vi "RELATORIO2LABVIEW.vi"() -> ()   [LabVIEW 2019]
uses:
  <vilib>/Instr/_visa.llb/VISA Configure Serial Port (Instr).vi
  <vilib>/express/express analysis/Spectral/Block/exnSpectralBlock spectral measurements RMS poly.vi
  <vilib>/express/express analysis/Spectral/Block/exnSpectralBlock spectral measurements RMS WFM.vi
  <vilib>/express/express analysis/Spectral/XNode/ExpressSpectralMeasurementsBlockNode.xnode
panel:
  out "Si":bool
  out "Lá":bool
  out "Sol":bool
  out "Fá":bool
  out "Mi":bool
  out "Ré":bool
  out "Dó":bool
  out "Análise espectral da onda - FFT (RMS)":cluster{"f0":dbl, "df":dbl, "magnitude":dbl[]}(graph)
  out "Amplitude do sinal (v) x tempo (s):":waveform(dbl)(graph)
  in  "Parar":bool
  out "Número de \nAmostras":u32 caption="Número de Amostras"
  in  "Número de Blocos de Dados":u32=100 min=1 max=50000 step=1
  in  "Frequencia de Amostragem":dbl=75000.0
  in  "VCC":dbl=5.0
  in  "Resolução":i16=8
  in  "COM Port":refnum<visa-resource-name>
  in  "Baudrate":u32=2000000
  # "PSI3214 - Turma 6\nAntonio Oliveira Pedroso da Cruz — 11798787\nDaniel Martins Cabanas — 12486742\nJoão Pedro Lima A. de Carvalho — 11260846"
  # "Notas musicais"
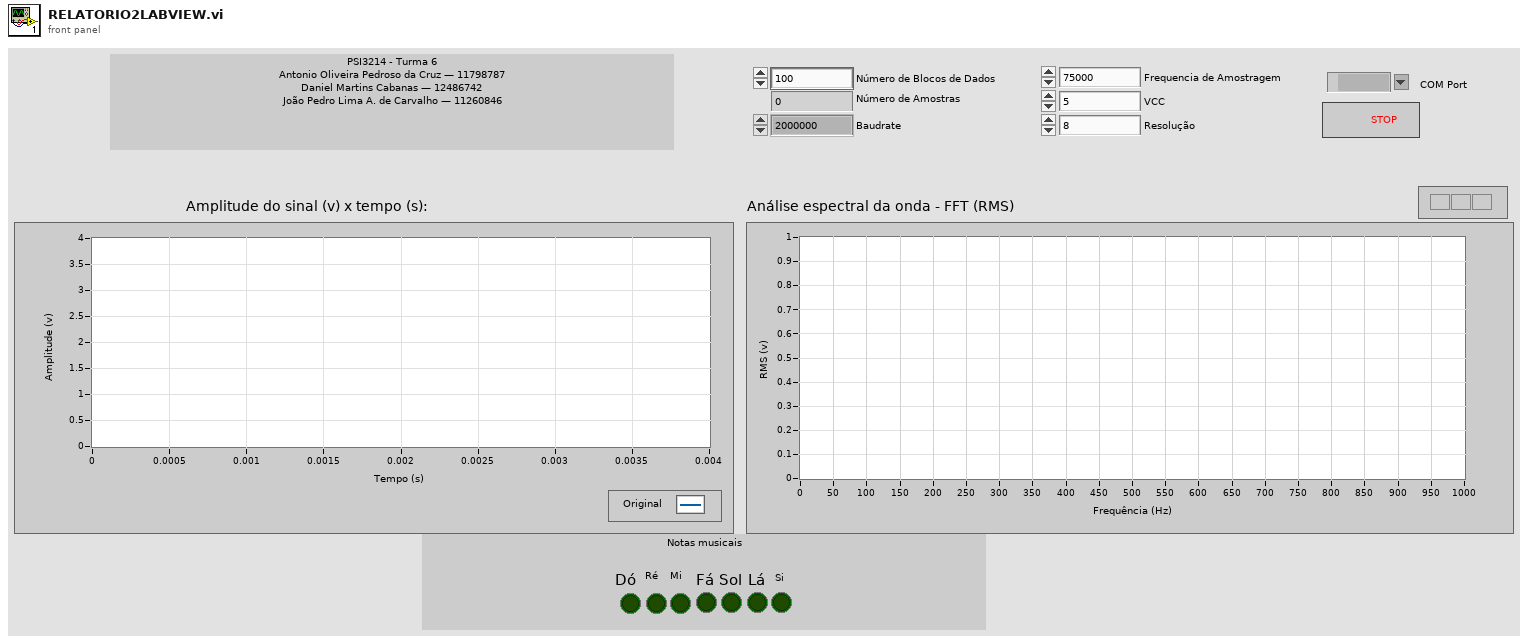
[diagram p1: front panel]
types:
  T1 = cluster{"averaging mode":u16, "weighting mode":u16, "number of averages":u32}
  T2 = cluster{"dB On (F)":bool, "unwrap phase (F)":bool, "convert to degree (F)":bool}
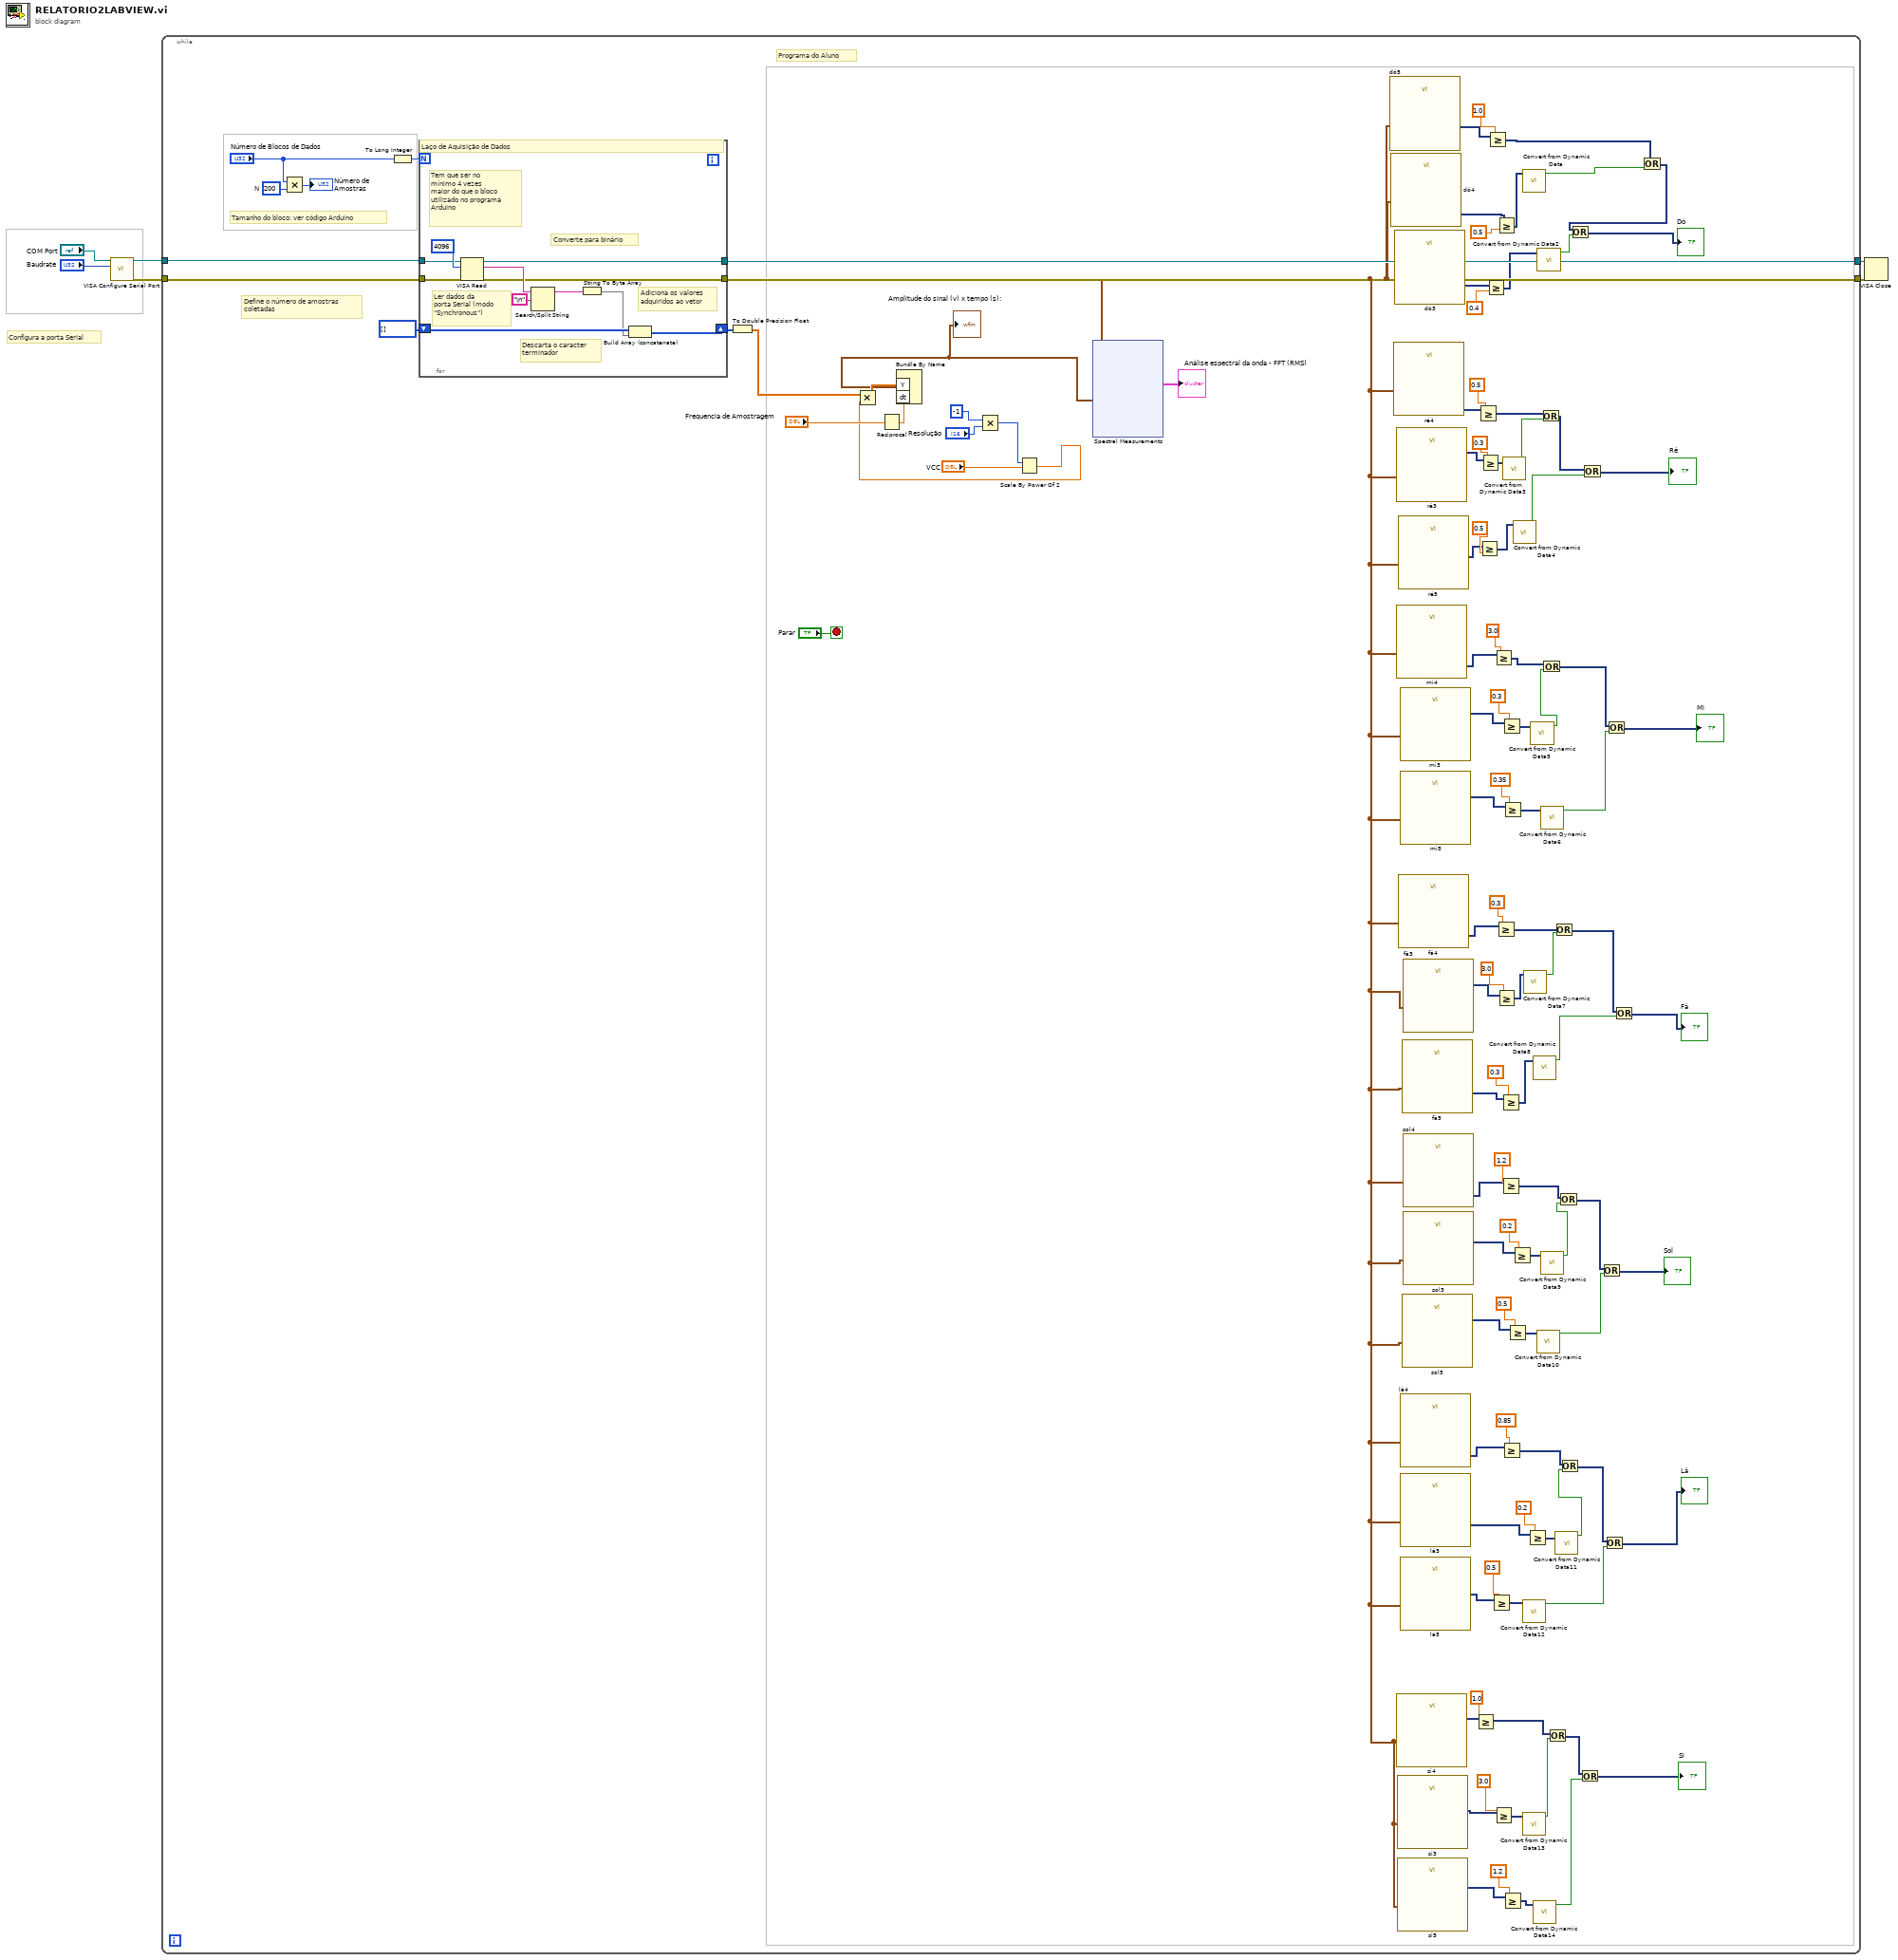
[diagram p0: block diagram]
diagram:
  # "Configura a porta Serial"
  n1 = call-poly "VISA Configure Serial Port"("VISA resource name"="COM Port", "baud rate (9600)"="Baudrate") -> ("VISA resource name out"=w4:refnum<visa-resource-name>, "error out"=w3:errorcluster)  [unwired: 12 in]
  n2 = while {
    tunnel: w4 -> [w119]
    tunnel: w3 -> [w118]
    tunnel: [w117] -> w2
    tunnel: [w116] -> w1
    stop <- "Parar" stop-if-true
    w110 = u32 200  # N
    # "Programa do Aluno"
    # "Tamanho do bloco: ver código Arduino"
    # "Define o número de amostras \ncoletadas"
    n3 = Multiply(x="Número de Blocos de Dados", y=w110) -> (x*y=→"Número de \nAmostras":u32)
    n4 = To Long Integer(number="Número de Blocos de Dados") -> (32bit integer=w113:i32)
    n5 = for {
      N: w113 -> [_]
      tunnel: w119 -> [w136]
      tunnel: w118 -> [w135]
      tunnel: [w134] -> w117
      tunnel: [w133] -> w116
      shift-right: [w130] -> w109
      shift-left: u8[] [] -> [w132]
      # "Adiciona os valores\nadquiridos ao vetor"
      # "Converte para binário"
      # "Descarta o caracter\nterminador"
      # "Ler dados da\nporta Serial (modo \"Synchronous\")"
      # "Tem que ser no \nmínimo 4 vezes \nmaior do que o bloco\nutilizado no programa \nArduino"
      # "Laço de Aquisição de Dados"
      n6 = VISA Read(VISA resource name=w136, byte count=u32 4096, error in (no error)=w135) -> (VISA resource name out=w134:refnum<visa-resource-name>, read buffer=w138:string, error out=w133:errorcluster)  [unwired: 1 out]
      n7 = Search/Split String(string=w138, search string/char (-)="\n") -> (substring before match=w140:string)  [unwired: 1 in, 2 out]
      n8 = String To Byte Array(string=w140) -> (unsigned byte array=w131:u8[])
      n9 = Build Array (concatenate)(w132, w131) -> (w130:u8[])
    }
    n10 = To Double Precision Float(number=w109) -> (double precision float=w108:dbl[])
    n11 = Reciprocal(x="Frequencia de Amostragem") -> (1/x=w100:dbl)
    n12 = Multiply(x=-1, y="Resolução") -> (x*y=w103:i32)
    n13 = Scale By Power Of 2(n=w103, x="VCC") -> (x*2^n=w8:dbl)
    n14 = Multiply(x=w108, y=w8) -> (x*y=w107:dbl[])
    n15 = Bundle By Name("Y"=w107, "dt"=w100) -> (w9:waveform(dbl))  [unwired: 1 in]
    "Amplitude do sinal (v) x tempo (s):" <- w9
    n16 = xnode "Spectral Measurements"("Signals"=w9) -> ("FFT - (RMS)"=→"Análise espectral da onda - FFT (RMS)":cluster{"f0":dbl, "df":dbl, "magnitude":dbl[]})  [unwired: 1 in, 2 out]
    n17 = call "dó5"("Signal"=w9) -> ("Filtered Signal"=w84:dynamicdata)  [unwired: 9 in, 1 out]
    n18 = call "dó4"("Signal"=w9) -> ("Filtered Signal"=w59:dynamicdata)  [unwired: 9 in, 1 out]
    n19 = call "ré4"("Signal"=w9) -> ("Filtered Signal"=w91:dynamicdata)  [unwired: 9 in, 1 out]
    n20 = call "dó3"("Signal"=w9) -> ("Filtered Signal"=w98:dynamicdata)  [unwired: 9 in, 1 out]
    n21 = call "ré3"("Signal"=w9) -> ("Filtered Signal"=w82:dynamicdata)  [unwired: 9 in, 1 out]
    n22 = call "mi4"("Signal"=w9) -> ("Filtered Signal"=w90:dynamicdata)  [unwired: 9 in, 1 out]
    n23 = call "si4"("Signal"=w9) -> ("Filtered Signal"=w86:dynamicdata)  [unwired: 9 in, 1 out]
    n24 = call "si3"("Signal"=w9) -> ("Filtered Signal"=w62:dynamicdata)  [unwired: 9 in, 1 out]
    n25 = call "si5"("Signal"=w9) -> ("Filtered Signal"=w60:dynamicdata)  [unwired: 9 in, 1 out]
    n26 = call "ré5"("Signal"=w9) -> ("Filtered Signal"=w80:dynamicdata)  [unwired: 9 in, 1 out]
    n27 = call "fá4"("Signal"=w9) -> ("Filtered Signal"=w89:dynamicdata)  [unwired: 9 in, 1 out]
    n28 = call "mi3"("Signal"=w9) -> ("Filtered Signal"=w78:dynamicdata)  [unwired: 9 in, 1 out]
    n29 = call "lá4"("Signal"=w9) -> ("Filtered Signal"=w87:dynamicdata)  [unwired: 9 in, 1 out]
    n30 = call "lá3"("Signal"=w9) -> ("Filtered Signal"=w66:dynamicdata)  [unwired: 9 in, 1 out]
    n31 = call "lá5"("Signal"=w9) -> ("Filtered Signal"=w64:dynamicdata)  [unwired: 9 in, 1 out]
    n32 = call "mi5"("Signal"=w9) -> ("Filtered Signal"=w76:dynamicdata)  [unwired: 9 in, 1 out]
    n33 = call "fá5"("Signal"=w9) -> ("Filtered Signal"=w72:dynamicdata)  [unwired: 9 in, 1 out]
    n34 = call "sol5"("Signal"=w9) -> ("Filtered Signal"=w68:dynamicdata)  [unwired: 9 in, 1 out]
    n35 = call "sol3"("Signal"=w9) -> ("Filtered Signal"=w70:dynamicdata)  [unwired: 9 in, 1 out]
    n36 = call "fá3"("Signal"=w9) -> ("Filtered Signal"=w74:dynamicdata)  [unwired: 9 in, 1 out]
    n37 = call "sol4"("Signal"=w9) -> ("Filtered Signal"=w88:dynamicdata)  [unwired: 9 in, 1 out]
    n38 = Greater Or Equal?(x=w86, y=1.0) -> (x >= y?=w15:dynamicdata)
    n39 = Greater Or Equal?(x=w91, y=0.5) -> (x >= y?=w49:dynamicdata)
    n40 = Greater Or Equal?(x=w80, y=0.5) -> (x >= y?=w48:dynamicdata)
    n41 = Greater Or Equal?(x=w82, y=0.3) -> (x >= y?=w50:dynamicdata)
    n42 = Greater Or Equal?(x=w98, y=0.4) -> (x >= y?=w53:dynamicdata)
    n43 = Greater Or Equal?(x=w84, y=1.0) -> (x >= y?=w57:dynamicdata)
    n44 = Greater Or Equal?(x=w64, y=0.5) -> (x >= y?=w20:dynamicdata)
    n45 = Greater Or Equal?(x=w90, y=3.0) -> (x >= y?=w43:dynamicdata)
    n46 = Greater Or Equal?(x=w62, y=3.0) -> (x >= y?=w16:dynamicdata)
    n47 = Greater Or Equal?(x=w89, y=0.3) -> (x >= y?=w36:dynamicdata)
    n48 = Greater Or Equal?(x=w59, y=0.5) -> (x >= y?=w55:dynamicdata)
    n49 = Greater Or Equal?(x=w74, y=3.0) -> (x >= y?=w37:dynamicdata)
    n50 = Greater Or Equal?(x=w72, y=0.3) -> (x >= y?=w34:dynamicdata)
    n51 = Greater Or Equal?(x=w88, y=1.2) -> (x >= y?=w29:dynamicdata)
    n52 = Greater Or Equal?(x=w78, y=0.3) -> (x >= y?=w44:dynamicdata)
    n53 = Greater Or Equal?(x=w87, y=0.85) -> (x >= y?=w22:dynamicdata)
    n54 = Greater Or Equal?(x=w76, y=0.35) -> (x >= y?=w41:dynamicdata)
    n55 = Greater Or Equal?(x=w60, y=1.2) -> (x >= y?=w13:dynamicdata)
    n56 = call "Convert from Dynamic Data3"("Dynamic Data Type"=w50) -> ("Scalar"=w7:bool)  [unwired: 3 in]
    n57 = Greater Or Equal?(x=w68, y=0.5) -> (x >= y?=w27:dynamicdata)
    n58 = Greater Or Equal?(x=w70, y=0.2) -> (x >= y?=w30:dynamicdata)
    n59 = call "Convert from Dynamic Data4"("Dynamic Data Type"=w48) -> ("Scalar"=w47:bool)  [unwired: 3 in]
    n60 = call "Convert from Dynamic Data"("Dynamic Data Type"=w55) -> ("Scalar"=w56:bool)  [unwired: 3 in]
    n61 = call "Convert from Dynamic Data12"("Dynamic Data Type"=w20) -> ("Scalar"=w18:bool)  [unwired: 3 in]
    n62 = call "Convert from Dynamic Data13"("Dynamic Data Type"=w16) -> ("Scalar"=w14:bool)  [unwired: 3 in]
    n63 = call "Convert from Dynamic Data7"("Dynamic Data Type"=w37) -> ("Scalar"=w35:bool)  [unwired: 3 in]
    n64 = Greater Or Equal?(x=w66, y=0.2) -> (x >= y?=w23:dynamicdata)
    n65 = call "Convert from Dynamic Data5"("Dynamic Data Type"=w44) -> ("Scalar"=w42:bool)  [unwired: 3 in]
    n66 = call "Convert from Dynamic Data8"("Dynamic Data Type"=w34) -> ("Scalar"=w33:bool)  [unwired: 3 in]
    n67 = call "Convert from Dynamic Data14"("Dynamic Data Type"=w13) -> ("Scalar"=w12:bool)  [unwired: 3 in]
    n68 = call "Convert from Dynamic Data10"("Dynamic Data Type"=w27) -> ("Scalar"=w25:bool)  [unwired: 3 in]
    n69 = call "Convert from Dynamic Data2"("Dynamic Data Type"=w53) -> ("Scalar"=w52:bool)  [unwired: 3 in]
    n70 = Or(x=w49, y=w7) -> (x .or. y?=w46:dynamicdata)
    n71 = Or(x=w43, y=w42) -> (x .or. y?=w40:dynamicdata)
    n72 = call "Convert from Dynamic Data6"("Dynamic Data Type"=w41) -> ("Scalar"=w39:bool)  [unwired: 3 in]
    n73 = call "Convert from Dynamic Data9"("Dynamic Data Type"=w30) -> ("Scalar"=w28:bool)  [unwired: 3 in]
    n74 = Or(x=w15, y=w14) -> (x .or. y?=w11:dynamicdata)
    n75 = Or(x=w36, y=w35) -> (x .or. y?=w32:dynamicdata)
    n76 = call "Convert from Dynamic Data11"("Dynamic Data Type"=w23) -> ("Scalar"=w21:bool)  [unwired: 3 in]
    n77 = Or(x=w29, y=w28) -> (x .or. y?=w26:dynamicdata)
    n78 = Or(x=w22, y=w21) -> (x .or. y?=w19:dynamicdata)
    n79 = Or(x=w11, y=w12) -> (x .or. y?=→"Si":dynamicdata)
    n80 = Or(x=w46, y=w47) -> (x .or. y?=→"Ré":dynamicdata)
    n81 = Or(x=w26, y=w25) -> (x .or. y?=→"Sol":dynamicdata)
    n82 = Or(x=w19, y=w18) -> (x .or. y?=→"Lá":dynamicdata)
    n83 = Or(x=w40, y=w39) -> (x .or. y?=→"Mi":dynamicdata)
    n84 = Or(x=w32, y=w33) -> (x .or. y?=→"Fá":dynamicdata)
    n85 = Or(x=w57, y=w56) -> (x .or. y?=w54:dynamicdata)
    n86 = Or(x=w54, y=w52) -> (x .or. y?=→"Dó":dynamicdata)
  }
  n87 = VISA Close(VISA resource name=w2, error in (no error)=w1) -> ()  [unwired: 1 out]
